vi "U8_Array_to_graph.vi"(10 "Array In":u8[](array[numeric]), 11 "Nmbr_of_datasamples":dbl=128.0) -> (1 "mV":dbl, 2 "Waveform Graph":dbl[](graph), 3 "Loop count":dbl)   [LabVIEW 2012]
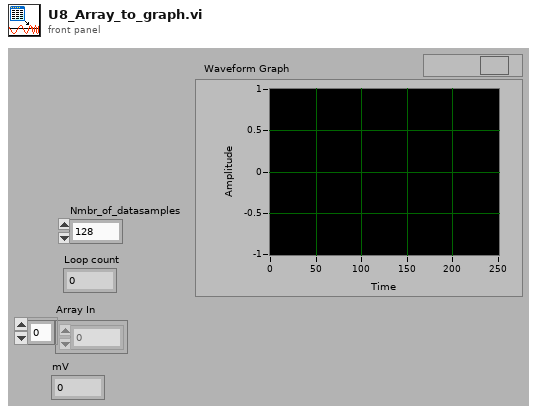
[diagram p1: front panel]
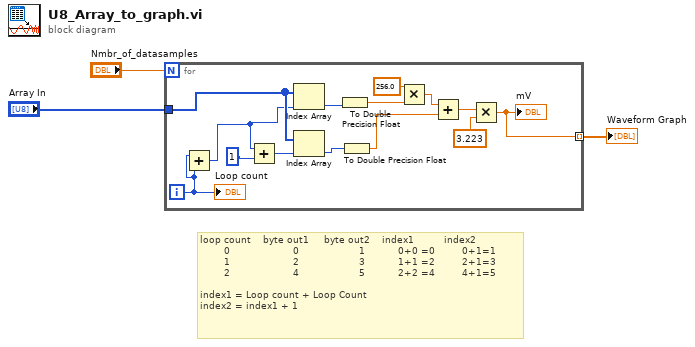
[diagram p0: block diagram]
diagram:
  # "loop count    byte out1     byte out2    index1          index2         \n        0                     0                    1           0+0 =0         0+1=1\n        1                     2                    3           1+1 =2         2+1=3\n        2                     4                    5           2+2 =4         4+1=5\n\nindex1 = Loop count + Loop Count\nindex2 = index1 + 1"
  n1 = for {
    N: "Nmbr_of_datasamples" -> [_]
    tunnel: [w9] -> w3 mode=indexing
    tunnel: "Array In" -> [w6]
    i -> [w5]
    n2 = Add(x=w5, y=w5) -> (x+y=w4:i32)
    n3 = Add(x=w4, y=1) -> (x+y=w10:i32)
    n4 = Index Array(array=w6, index=w4) -> (element=w8:u8)
    n5 = Index Array(array=w6, index=w10) -> (element=w7:u8)
    n6 = To Double Precision Float(number=w8) -> (double precision float=w16:dbl)
    n7 = To Double Precision Float(number=w7) -> (double precision float=w17:dbl)
    n8 = Multiply(x=256.0, y=w16) -> (x*y=w13:dbl)
    n9 = Add(x=w13, y=w17) -> (x+y=w14:dbl)
    n10 = Multiply(x=w14, y=3.223) -> (x*y=w9:dbl)
    "mV" <- w9
    "Loop count" <- w5
  }
  "Waveform Graph" <- w3
